vi "HFRR ADV v08.vi"() -> ()   [LabVIEW 2025] (continued)
        stop <- w5093 stop-if-true
        n3621 = local read "powstat"() -> (w5094:bool)
        n3622 = case shown="True" w5094 {
          frame False {
          }
          frame True {
            n3623 = local read "RUN"() -> (w5097:bool)
            n3624 = case shown="True" w5097 {
              frame False {
                w5127 = 65.0 ("y")
                n3625 = local read "Set Hz"() -> (w5155:dbl)
                n3626 = local read "NORMAL LOAD"() -> (w5156:dbl)
                n3627 = Multiply(x=w5155, y=60.0) -> (x*y=w5162:dbl)
                n3628 = Multiply(x=1.2 ("y"), y=0.949) -> (x*y=w5131:dbl)
                n3629 = Multiply(x=1.2 ("y"), y=0.8166) -> (x*y=w5135:dbl)
                n3630 = Multiply(x=1.2 ("y"), y=0.851) -> (x*y=w5130:dbl)
                n3631 = local read "FF 2"() -> (w5154:dbl)
                n3632 = Absolute Value(x=w5162) -> (abs(x)=w5160:dbl)
                n3633 = local read "Stroke"() -> (w5129:dbl)
                n3634 = Less?(x=w5129, y=w5135) -> (x < y?=w5132:bool)
                n3635 = In Range and Coerce(upper limit=w5131, x=w5129, lower limit=w5130) -> (In Range?=w5133:bool)  [unwired: 1 out]
                n3636 = case shown="13.." w5154 {
                  tunnel: [1 2 3] -> w5152
                  frame 0..10, Default {
                    # "Normal"
                  }
                  frame 11, 12 {
                  }
                  frame 13.. {
                  }
                }
                "FF STATE" <- w5152
                n3637 = local read "TEMP"() -> (w5115:dbl)
                n3638 = case shown="3601.." w5160 {
                  tunnel: [1 2 3] -> w5158
                  frame 0..3000, Default {
                    # "Normal"
                  }
                  frame 3001..3600 {
                  }
                  frame 3601.. {
                  }
                }
                n3639 = case shown="11.." w5156 {
                  tunnel: [1 3] -> w5157
                  frame 1..10, Default {
                  }
                  frame 11.. {
                  }
                }
                "NL STATE" <- w5157
                n3640 = Multiply(x=1.2 ("y"), y=0.95) -> (x*y=w5145:dbl)
                n3641 = Multiply(x=w5127, y=0.954) -> (x*y=w5119:dbl)
                n3642 = Or(x=w5132, y=w5133) -> (x .or. y?=w5134:bool)
                n3643 = Greater Or Equal?(x=w5129, y=w5145) -> (x >= y?=w5142:bool)
                n3644 = Multiply(x=w5127, y=0.99) -> (x*y=w5116:dbl)
                n3645 = Greater Or Equal?(x=w5115, y=w5116) -> (x >= y?=w5121:bool)
                n3646 = Greater Or Equal?(x=w5115, y=w5119) -> (x >= y?=w5118:bool)
                n3647 = case shown="0, 1, Default" w5129 {
                  tunnel: [1 3] -> w5146
                  frame 0, 1, Default {
                  }
                  frame 2.. {
                  }
                }
                n3648 = case shown="True" w5142 {
                  tunnel: [1 3] -> w5147
                  frame False {
                  }
                  frame True {
                  }
                }
                n3649 = case shown="True" w5134 {
                  tunnel: [1 2] -> w5148
                  frame False {
                  }
                  frame True {
                  }
                }
                n3650 = case shown="..0" w5115 {
                  tunnel: [2 3 3 1] -> w5122
                  frame 61, 62 {
                  }
                  frame 63.. {
                  }
                  frame ..0 {
                  }
                  frame 10..60, Default {
                  }
                }
                n3651 = case shown="True" w5121 {
                  tunnel: [1 3] -> w5123
                  frame False {
                  }
                  frame True {
                  }
                }
                n3652 = Number To Decimal String(number=w5158) -> (decimal integer string=w5159:string)  [unwired: 1 in]
                n3653 = case shown="True" w5118 {
                  tunnel: [1 2] -> w5124
                  frame False {
                  }
                  frame True {
                  }
                }
                n3654 = Number To Decimal String(number=1) -> (decimal integer string=→"Air temp":string)  [unwired: 1 in]
                n3655 = Number To Decimal String(number=w5152) -> (decimal integer string=→"ff_st":string)  [unwired: 1 in]
                n3656 = local write "sp_st"(w5159) -> ()
                n3657 = Number To Decimal String(number=w5157) -> (decimal integer string=→"nl_st":string)  [unwired: 1 in]
                n3658 = Build Array(w5122, w5123, w5124) -> (w5125:i32[])
                n3659 = Build Array(w5146, w5147, w5148) -> (w5149:i32[])
                n3660 = Array Max & Min(array=w5125) -> (max value=w5126:i32)  [unwired: 3 out]
                n3661 = Array Max & Min(array=w5149) -> (max value=w5150:i32)  [unwired: 3 out]
                n3662 = Number To Decimal String(number=w5126) -> (decimal integer string=w5114:string)  [unwired: 1 in]
                n3663 = Number To Decimal String(number=w5150) -> (decimal integer string=→"Stroke Ln 2":string)  [unwired: 1 in]
                n3664 = local write "temp_st"(w5114) -> ()
              }
              frame True {
                w5212 = 65.0 ("y")
                # "Healthy -1\nWarning -2\nError -3"
                n3665 = local read "TEMP"() -> (w5223:dbl)
                n3666 = local read "NORMAL LOAD"() -> (w5227:dbl)
                n3667 = local read "Set Hz"() -> (w5225:dbl)
                n3668 = Multiply(x=1.2 ("y"), y=0.949) -> (x*y=w5207:dbl)
                n3669 = Multiply(x=1.2 ("y"), y=0.8166) -> (x*y=w5203:dbl)
                n3670 = Multiply(x=1.2 ("y"), y=0.851) -> (x*y=w5208:dbl)
                n3671 = Multiply(x=w5212, y=0.954) -> (x*y=w5219:dbl)
                n3672 = Multiply(x=w5212, y=0.99) -> (x*y=w5222:dbl)
                n3673 = Greater Or Equal?(x=w5223, y=w5222) -> (x >= y?=w5217:bool)
                n3674 = Multiply(x=w5225, y=60.0) -> (x*y=w5231:dbl)
                n3675 = Greater Or Equal?(x=w5223, y=w5219) -> (x >= y?=w5220:bool)
                n3676 = local read "FF 2"() -> (w5226:dbl)
                n3677 = local read "Stroke"() -> (w5209:dbl)
                n3678 = Less?(x=w5209, y=w5203) -> (x < y?=w5206:bool)
                n3679 = In Range and Coerce(upper limit=w5207, x=w5209, lower limit=w5208) -> (In Range?=w5205:bool)  [unwired: 1 out]
                n3680 = Absolute Value(x=w5231) -> (abs(x)=w5229:dbl)
                n3681 = case shown="63.." w5223 {
                  tunnel: [2 3 3 1] -> w5216
                  frame 61, 62 {
                  }
                  frame 63.. {
                  }
                  frame ..0 {
                  }
                  frame 10..60, Default {
                  }
                }
                n3682 = case shown="True" w5217 {
                  tunnel: [1 3] -> w5215
                  frame False {
                  }
                  frame True {
                  }
                }
                n3683 = case shown="True" w5220 {
                  tunnel: [1 2] -> w5214
                  frame False {
                  }
                  frame True {
                  }
                }
                n3684 = Multiply(x=1.2 ("y"), y=0.95) -> (x*y=w5193:dbl)
                n3685 = case shown="1..10, Default" w5227 {
                  tunnel: [1 3] -> w5234
                  frame 1..10, Default {
                  }
                  frame 11.. {
                  }
                }
                n3686 = case shown="0..10, Default" w5226 {
                  tunnel: [1 2 3] -> w5233
                  frame 0..10, Default {
                  }
                  frame 11, 12 {
                  }
                  frame 13.. {
                  }
                }
                n3687 = case shown="3601.." w5229 {
                  tunnel: [1 2 3] -> w5228
                  frame 0..3000, Default {
                    # "Normal"
                  }
                  frame 3001..3600 {
                  }
                  frame 3601.. {
                  }
                }
                n3688 = Or(x=w5206, y=w5205) -> (x .or. y?=w5204:bool)
                n3689 = Greater Or Equal?(x=w5209, y=w5193) -> (x >= y?=w5196:bool)
                n3690 = case shown="0, 1, Default" w5209 {
                  tunnel: [1 3] -> w5192
                  frame 0, 1, Default {
                  }
                  frame 2.. {
                  }
                }
                n3691 = case shown="True" w5196 {
                  tunnel: [1 3] -> w5191
                  frame False {
                  }
                  frame True {
                  }
                }
                n3692 = case shown="True" w5204 {
                  tunnel: [1 2] -> w5190
                  frame False {
                  }
                  frame True {
                  }
                }
                n3693 = Build Array(w5216, w5215, w5214) -> (w5213:i32[])
                n3694 = Number To Decimal String(number=w5228) -> (decimal integer string=→"sp_st":string)  [unwired: 1 in]
                n3695 = Array Max & Min(array=w5213) -> (max value=w5210:i32)  [unwired: 3 out]
                "TEMP STATE" <- w5210
                n3696 = Number To Decimal String(number=w5234) -> (decimal integer string=w5237:string)  [unwired: 1 in]
                n3697 = Number To Decimal String(number=w5233) -> (decimal integer string=w5235:string)  [unwired: 1 in]
                n3698 = Number To Decimal String(number=w5210) -> (decimal integer string=→"temp_st":string)  [unwired: 1 in]
                n3699 = Build Array(w5192, w5191, w5190) -> (w5189:i32[])
                n3700 = local write "nl_st"(w5237) -> ()
                n3701 = local write "ff_st"(w5235) -> ()
                n3702 = Number To Decimal String(number=1) -> (decimal integer string=w5232:string)  [unwired: 1 in]
                n3703 = Array Max & Min(array=w5189) -> (max value=w5188:i32)  [unwired: 3 out]
                n3704 = local write "Air temp"(w5232) -> ()
                n3705 = Number To Decimal String(number=w5188) -> (decimal integer string=w5187:string)  [unwired: 1 in]
                n3706 = local write "Stroke Ln 2"(w5187) -> ()
              }
            }
            n3707 = local read "Stroke Ln 2"() -> (w5099:string)
            n3708 = local read "nl_st"() -> (w5105:string)
            n3709 = local read "ff_st"() -> (w5102:string)
            n3710 = local read "sp_st"() -> (w5103:string)
            n3711 = local read "temp_st"() -> (w5104:string)
            n3712 = local read "Air temp"() -> (w5098:string)
            n3713 = Replace Array Subset(array="in", new element #1=w5105, index #1=1 ("index"), new element #2=w5102, index #2=2 ("index"), new element #3=w5104, index #3=3 ("index"), new element #4=w5103, index #4=4 ("index"), new element #5=w5099, index #5=5 ("index"), new element #6=w5098, index #6=6 ("index"), new element #7="Sensor State" ("new element/subarray"), index #7=0 ("index")) -> (→"out":string[])
          }
        }
        n3714 = Wait (ms)(milliseconds to wait=u32 10) -> ()  [unwired: 1 out]
        n3715 = local read "Quit"() -> (w5093:bool)
      }
      n3716 = while {
        stop <- w5068 stop-if-true
        n3717 = local read "run replace"() -> (w5070:bool)
        n3718 = Wait (ms)(milliseconds to wait=u32 100) -> ()  [unwired: 1 out]
        n3719 = Equal?(x="FLAG 2", y=0.0) -> (x = y?=w5071:bool)
        n3720 = case shown="True" w5071 {
          frame False {
          }
          frame True {
            n3721 = local write "FLAG 2"(100.0 ("FLAG 2")) -> ()
            n3722 = call <vilib>:"Read Characters From File.vi"("file path (dialog if empty)"=path "C:/LAB-IQ-NXT/WO 2449 TT.sig", "convert eol? (no:F)"=FALSE ("append to file? (new file:F)")) -> ("character string"=w5074:string)  [unwired: 4 in, 3 out]
            n3723 = call <vilib>:"Read Characters From File.vi"("file path (dialog if empty)"=path "C:/LAB-IQ-NXT/WO 2449 TRH.sig", "convert eol? (no:F)"=FALSE ("append to file? (new file:F)")) -> ("character string"=w5075:string)  [unwired: 4 in, 3 out]
            n3724 = Decimal String To Number(string=w5074) -> (number=w5076:i32)  [unwired: 2 in, 1 out]
            n3725 = local write "Total No. of Tests"(w5076) -> ()
            n3726 = Decimal String To Number(string=w5075) -> (number=w5079:i32)  [unwired: 2 in, 1 out]
            n3727 = local write "SEN.RUN HRS"(w5079) -> ()
          }
        }
        n3728 = case shown="True" w5070 {
          frame False {
          }
          frame True {
            n3729 = Equal?(x="FLAG 4", y=0.0) -> (x = y?=w5083:bool)
            n3730 = case shown="False" w5083 {
              frame False {
                n3731 = Get Date/Time In Seconds() -> (seconds since 1Jan1904=w5089:timestamp)
                n3732 = local read "START 3"() -> (w5087:dbl)
                n3733 = To Double Precision Float(number=w5089) -> (double precision float=w5088:dbl)
                n3734 = Subtract(x=w5088, y=w5087) -> (x-y=→"SENSOR TIME":dbl)
              }
              frame True {
                n3735 = Get Date/Time In Seconds() -> (seconds since 1Jan1904=w5091:timestamp)
                n3736 = local write "FLAG 4"(100.0 ("FLAG")) -> ()
                n3737 = To Double Precision Float(number=w5091) -> (double precision float=→"START 3":dbl)
              }
            }
          }
        }
        n3738 = local read "Quit"() -> (w5068:bool)
      }
      n3739 = while {
        shift-right: [w4868] -> _
        shift-left: _ -> [w4869]
        tunnel: [w4864] -> _
        i -> [w4864]
        stop <- w4863 stop-if-true
        n3740 = Wait (ms)(milliseconds to wait=u32 50 ("Refresh Rate (ms)")) -> ()  [unwired: 1 out]
        n3741 = local read "Json End Flg"() -> (w4865:bool)
        n3742 = Not(x="Upld AR 2") -> ()  [unwired: 1 out]
        n3743 = local read "Upld AR 2"() -> (w4866:bool)
        n3744 = call "Elapsed Time9"("Time Target (s)"="Sen.Upload Rate (s)", "Reset"=FALSE, "Auto Reset"=TRUE) -> ("Time has Elapsed"=w4875:bool)  [unwired: 9 in, 7 out]
        n3745 = Or(x=w4875, y=w4865) -> (x .or. y?=w4871:bool)
        n3746 = case shown="True" w4871 {
          frame False {
          }
          frame True {
            w4967 = "\"SensorName\":\"" ("string")
            w4937 = " \"},{"
            w4962 = "\",\"SensorState\":\""
            w4964 = "\",\"SensorModelNumber\":\"" ("string")
            w4963 = "\",\"SensorRuntimeHours\":\"" ("string")
            n3747 = local read "model num"() -> (w4961:string[])
            n3748 = local read "Sensor name"() -> (w4980:string[])
            n3749 = local read "run"() -> (w4951:string[])
            n3750 = local read "SENSOR TIME"() -> (w4907:dbl)
            n3751 = local read "out"() -> (w4900:string[])
            n3752 = local read "Total No. of Tests"() -> (w4905:dbl)
            n3753 = Select(t=60.0, s="Run test 3", f=3600.0) -> (s? t:f=w4915:dbl)
            n3754 = Index Array(array=w4961, index #1=1 ("index")) -> (element #1=w4960:string, element #2=w4959:string, element #3=w4958:string, element #4=w4957:string, element #5=w4956:string, element #6=w4955:string)  [unwired: 5 in]
            n3755 = Index Array(array=w4951, index #1=1 ("index")) -> (element #1=w4950:string, element #2=w4949:string, element #3=w4948:string, element #4=w4947:string, element #5=w4946:string, element #6=w4945:string)  [unwired: 5 in]
            n3756 = Index Array(array=w4980, index #1=1 ("index")) -> (element #1=w4979:string, element #2=w4978:string, element #3=w4977:string, element #4=w4976:string, element #5=w4966:string, element #6=w4965:string)  [unwired: 5 in]
            n3757 = Index Array(array=w4900, index #1=1 ("index")) -> (element #1=w4932:string, element #2=w4931:string, element #3=w4930:string, element #4=w4929:string, element #5=w4928:string, element #6=w4927:string)  [unwired: 5 in]
            n3758 = local read "SEN.RUN HRS"() -> (w4903:dbl)
            n3759 = Divide(x=w4907, y=w4915) -> (x/y=w4914:dbl)
            n3760 = Increment(x=w4914) -> (x+1=w4910:dbl)
            n3761 = Number To Decimal String(number=w4910) -> (decimal integer string=→"run hrs":string)  [unwired: 1 in]
            n3762 = Divide(x=w4903, y=3600.0 ("f")) -> (x/y=w4898:dbl)
            n3763 = Round To Nearest(number=w4898) -> (nearest integer value=w4896:dbl)
            n3764 = Number To Decimal String(number=w4896) -> (decimal integer string=w4897:string)  [unwired: 1 in]
            n3765 = Number To Decimal String(number=w4905) -> (decimal integer string=w4906:string)  [unwired: 1 in]
            n3766 = local read "Model No"() -> (w4911:string)
            n3767 = local read "UUID"() -> (w5006:string)
            n3768 = local read "Serial No"() -> (w5010:string)
            n3769 = local read "Secret Key"() -> (w5011:string)
            n3770 = Concatenate Strings("\",\"MachineSerialNumber\":\"" ("string"), w5010) -> (w5014:string)
            n3771 = Concatenate Strings("\",\"ModelNumber\":\"" ("string"), w4911) -> (w4912:string)
            n3772 = Concatenate Strings("\",\"MachineRuntimeHours\":\"" ("string"), w4897) -> (w5015:string)
            n3773 = Concatenate Strings("\",\"MachineRuntimeCycles\":\"", w4906) -> (w5008:string)
            n3774 = Concatenate Strings(w4964, w4960) -> (w4994:string)
            n3775 = Concatenate Strings(w4963, w4950) -> (w4995:string)
            n3776 = Concatenate Strings(w4962, w4932) -> (w4993:string)
            n3777 = Concatenate Strings(w5014, w4912, w5015, w5008) -> (w5017:string)
            n3778 = Concatenate Strings(w4964, w4959) -> (w4991:string)
            n3779 = Concatenate Strings(w4963, w4949) -> (w4990:string)
            n3780 = Concatenate Strings(w4962, w4931) -> (w4992:string)
            n3781 = Concatenate Strings(w4964, w4958) -> (w4986:string)
            n3782 = Concatenate Strings(w4963, w4948) -> (w4987:string)
            n3783 = Concatenate Strings(w4962, w4930) -> (w4985:string)
            n3784 = Concatenate Strings(w4964, w4957) -> (w4983:string)
            n3785 = Concatenate Strings(w4963, w4947) -> (w4982:string)
            n3786 = Concatenate Strings(w4962, w4929) -> (w4984:string)
            n3787 = Concatenate Strings(w4994, w4995, w4993) -> (w4996:string)
            n3788 = Concatenate Strings(w4964, w4956) -> (w4973:string)
            n3789 = Concatenate Strings(w4963, w4946) -> (w4974:string)
            n3790 = Concatenate Strings(w4964, w4955) -> (w4970:string)
            n3791 = Concatenate Strings(w4963, w4945) -> (w4969:string)
            n3792 = Concatenate Strings(w4962, w4928) -> (w4972:string)
            n3793 = Concatenate Strings(w4962, w4927) -> (w4971:string)
            n3794 = Concatenate Strings("{\"SecretKey\":\"", w5011, w5017, "\",\"UUID\" : \"", w5006, "\",\"SensorInformation\":", "[{" ("string")) -> (w4944:string)
            n3795 = Concatenate Strings(w4991, w4990, w4992) -> (w4989:string)
            n3796 = Concatenate Strings(w4986, w4987, w4985) -> (w4988:string)
            n3797 = Concatenate Strings(w4983, w4982, w4984) -> (w4981:string)
            n3798 = Concatenate Strings(w4973, w4974, w4972) -> (w4975:string)
            n3799 = Concatenate Strings(w4970, w4969, w4971) -> (w4968:string)
            n3800 = Concatenate Strings(w4967, w4979, w4996, w4937) -> (w4943:string)
            n3801 = Concatenate Strings(w4967, w4978, w4989, w4937) -> (w4942:string)
            n3802 = Concatenate Strings(w4967, w4977, w4988, w4937) -> (w4941:string)
            n3803 = Concatenate Strings(w4967, w4976, w4981, w4937) -> (w4940:string)
            n3804 = Concatenate Strings(w4967, w4966, w4975, w4937) -> (w4939:string)
            n3805 = Concatenate Strings(w4967, w4965, w4968, "\"}" ("string")) -> (w4938:string)
            n3806 = Concatenate Strings(w4944, w4943, w4942, w4941, w4940, w4939, w4938, "]}" ("string")) -> (w4935:string)
            n3807 = local read "SEN.RUN HRS"() -> (w4902:dbl)
            n3808 = disable-structure shown="Disabled" {
              frame Disabled {
                n3809 = local read "state"() -> (w5021:string[])
                n3810 = Delete From Array(array=w5021, index=0) -> (array with subset deleted=w5019:string[])  [unwired: 1 in, 1 out]
                n3811 = for {
                  N: 6 -> [_]
                  tunnel: w5019 -> [w5032] mode=indexing
                  tunnel: [w5031] -> w5018 mode=indexing
                  n3812 = Equal?(x=w5032, y="Warning") -> (x = y?=w5028:bool)
                  n3813 = Equal?(x=w5032, y="Healthy") -> (x = y?=w5025:bool)
                  n3814 = Select(t="2" ("y"), s=w5028, f="3" ("y")) -> (s? t:f=w5023:string)
                  n3815 = Select(t="1" ("y"), s=w5025, f=w5023) -> (s? t:f=w5031:string)
                }
                "state1" <- w5018
              }
              frame Enabled {
              }
            }
            n3816 = stacked-sequence {
              tunnel: w4935 -> [w5043 _ _]
              tunnel: [_ _ w5059] -> _
              frame #0 {
                (unwired) FALSE ("convert eol (F)")
                w5045 = enum16{"start", "end", "current"}."start" ("pos mode (0:2)")
                n3817 = local read "Path"() -> (w5039:path)
                n3818 = Path To String(path=w5039) -> (string=w5051:string)
                n3819 = Concatenate Strings(w5051, "\\", "Sensor File Name") -> (w5052:string)
                n3820 = local write "standard output 2"(" ") -> ()
                n3821 = String To Path(string=w5052) -> (path=w5042:path)
                n3822 = call <vilib>:"Open_Create_Replace File.vi"("advisory dialog? (display:T)"=FALSE, "function (open:0)"=T24."create or replace", "file path"=w5042) -> ("error out"=w5055:errorcluster, "refnum"=w5054:refnum<file>)  [unwired: 5 in, 2 out]
                n3823 = Set File Position(refnum=w5054, from (0:start)=w5045, error in=w5055) -> (refnum out=w5035:refnum<file>, error out=w5034:errorcluster)  [unwired: 1 in]
                n3824 = Write to Binary File(file (use dialog)=w5035, data=" ", error in=w5034, 5:FALSE ("prepend array or string size? (T)")) -> (refnum out=w5046:refnum<file>, error out=w5047:errorcluster)  [unwired: 2 in, 1 out]
                n3825 = Set File Position(offset (in bytes) (0)=w5045, refnum=w5046, error in=w5047) -> (refnum out=w5038:refnum<file>, error out=w5037:errorcluster)  [unwired: 1 in]
                n3826 = Write to Binary File(file (use dialog)=w5038, data=w5043, error in=w5037, 5:FALSE ("prepend array or string size? (T)")) -> (error out=w5041:errorcluster)  [unwired: 2 in, 2 out]
                n3827 = flat-sequence {
                  tunnel: w5042 -> [w5057]
                  tunnel: w5041 -> [_]
                  frame #0 {
                    n3828 = call <vilib>:"Read Characters From File.vi"("file path (dialog if empty)"=w5057) -> ("character string"=→"Sensor Health JSON string":string)  [unwired: 5 in, 3 out]
                  }
                }
                "SinglePoint  2" <- w5043
              }
              frame #1 {
              }
              frame #2 {
                (unwired) "\"Stored\": true" ("string")
                n3829 = call <vilib>:"System Exec.vi"("run minimized? (F)"=TRUE, "wait until completion? (T)"=TRUE, "working directory"=path "C:/LAB-IQ-NXT", "command line"="C:\\LAB-IQ-NXT\\JPostH.bat") -> ("standard error"=→"Respose From Server 2":string, "standard output"=w5062:string)  [unwired: 4 in, 2 out]
                "standard output 2" <- w5062
                n3830 = Match Pattern(string=w5062, regular expression="JSONH Check String") -> (match substring=w5060:string, offset past match=w5059:i32)  [unwired: 1 in, 2 out]
                n3831 = Equal?(x=w5060, y="JSONH Check String") -> (x = y?=→"Upload \nConfirmed 2":bool)
              }
            }
            n3832 = Divide(x=w4902, y=3600.0 ("f")) -> (x/y=w4895:dbl)
            n3833 = local read "run time"() -> (w4952:string[])
            n3834 = Round To Nearest(number=w4895) -> (nearest integer value=w4894:dbl)
            n3835 = Number To Decimal String(number=w4894) -> (decimal integer string=w4893:string)  [unwired: 1 in]
            n3836 = Index Array(array="Sensor Information", index (col) #1=0 ("disabled index (col)"), index (col) #2=1 ("index (col)"), index (col) #3=2 ("index (col)"), index (col) #4=3 ("index (col)")) -> (element #1=→"Sensor name":string[], element #2=→"model num":string[], element #3=→"run time":string[], element #4=→"state":string[])  [unwired: 4 in]
            n3837 = Insert Into Array(array=w4952, index=1, new element #1=w4893, new element #2=w4893, new element #3=w4893, new element #4=w4893, new element #5=w4893, new element #6=w4893) -> (w4917:string[])
            "run" <- w4917
            n3838 = local read "out"() -> (w4899:string[])
            n3839 = local read "Sensor Information"() -> (w4919:string[][])
            n3840 = Replace Array Subset(array=w4919, new element #1=w4917, index (col) #1=2 ("disabled index (col)"), new element #2=w4899, index (col) #2=3 ("index (col)")) -> (w4918:string[][])  [unwired: 2 in]
            n3841 = local write "Sensor Information"(w4918) -> ()
          }
        }
        n3842 = case shown="True" w4866 {
          frame False {
          }
          frame True {
            n3843 = Equal?(x="FLAG", y=0.0) -> (x = y?=w4883:bool)
            n3844 = case shown="False" w4883 {
              frame False {
                n3845 = Get Date/Time In Seconds() -> (seconds since 1Jan1904=w4889:timestamp)
                n3846 = local read "START 2"() -> (w4887:dbl)
                n3847 = To Double Precision Float(number=w4889) -> (double precision float=w4888:dbl)
                n3848 = Subtract(x=w4888, y=w4887) -> (x-y=→"SENSOR TIME  2":dbl)
              }
              frame True {
                n3849 = Get Date/Time In Seconds() -> (seconds since 1Jan1904=w4891:timestamp)
                n3850 = To Double Precision Float(number=w4891) -> (double precision float=→"START 2":dbl)
                n3851 = local write "FLAG"(100.0 ("FLAG")) -> ()
              }
            }
          }
        }
        n3852 = disable-structure shown="Disabled" {
          disable-tunnel: w4869 -> [w4878 _]
          disable-tunnel: [w4877 _] -> w4868
          frame Disabled {
            n3853 = local read "Json St Flg"() -> (w4876:bool)
            n3854 = case shown="True" w4876 {
              tunnel: w4878 -> [w4879 w4881]
              tunnel: [w4879 w4880] -> w4877
              frame False {
              }
              frame True {
                n3855 = Increment(x=w4881) -> (x+1=w4880:dbl)
                "T cycle" <- w4880
                n3856 = local write "Json St Flg"(FALSE ("Json St Flg")) -> ()
              }
            }
          }
          frame Enabled {
          }
        }
        n3857 = local read "Quit"() -> (w4863:bool)
      }
    }
    frame Enabled {
    }
  }
  n3858 = stacked-sequence {
    tunnel: [w5261] -> w28
    frame #0 {
      w5261 = FALSE ("Upload \nConfirmed")
      n3859 = local write "Upload \nConfirmed"(w5261) -> ()
      n3860 = local write "St Str"("") -> ()
    }
  }
  n3861 = disable-structure shown="Disabled" {
    disable-tunnel: w28 -> [w5262 _]
    frame Disabled {
      n3862 = case shown="True" {
        selector: _ -> [_ _]
        tunnel: w5262 -> [_ w5263]
        frame False {
        }
        frame True {
          n3863 = while {
            tunnel: [w5269] -> _
            tunnel: w5263 -> [_]
            i -> [w5269]
            stop <- w5264 stop-if-true
            n3864 = local read "Json End Flg"() -> (w5268:bool)
            n3865 = Wait (ms)(milliseconds to wait=u32 20 ("Refresh Rate (ms)")) -> ()  [unwired: 1 out]
            n3866 = local read "refresh flag"() -> (w5265:bool)
            n3867 = local read "RUN"() -> (w5266:bool)
            n3868 = And(x=w5266, y=w5265) -> (x .and. y?=w5267:bool)
            n3869 = Or(x=w5267, y=w5268) -> (x .or. y?=w5270:bool)
            "AR Led" <- w5270
            n3870 = case shown="True" w5270 {
              frame False {
              }
              frame True {
                w5287 = "\",\""
                n3871 = local read "UUID"() -> (w5285:string)
                n3872 = local write "refresh flag"(FALSE ("refresh flag")) -> ()
                n3873 = local read "time"() -> (w5274:dbl)
                n3874 = Multiply(x=w5274, y=60.0) -> (x*y=w5273:dbl)
                n3875 = Concatenate Strings("UUID\" : \"", w5285, "\"}") -> (w5288:string)
                n3876 = Number To Fractional String(number=w5273, width (-)=i16 10, precision (6)=i16 4) -> (F-format string=w5302:string)  [unwired: 1 in]
                n3877 = Concatenate Strings("{", "\"Time\":\"", w5302, w5287) -> (w5297:string)
                n3878 = stacked-sequence {
                  tunnel: w5287 -> [w5350 w5358 w5365 w5373 w5381 w5390 w5397]
                  tunnel: [w5351 _ _ _ _ _ _] -> w5301
                  tunnel: [_ w5359 _ _ _ _ _] -> w5300
                  tunnel: [_ _ w5366 _ _ _ _] -> w5299
                  tunnel: [_ _ _ w5375 _ _ _] -> w5298
                  tunnel: w5288 -> [_ _ _ _ _ _ w5408]
                  tunnel: [_ _ _ _ _ _ w5407] -> w5284
                  tunnel: [_ _ _ _ _ w5387 _] -> w5283
                  tunnel: [_ _ _ _ w5380 _ _] -> w5282
                  frame #0 {
                    n3879 = local read "NORMAL LOAD"() -> (w5349:dbl)
                    n3880 = Number To Fractional String(number=w5349, width (-)=i16 10, precision (6)=i16 4) -> (F-format string=w5352:string)  [unwired: 1 in]
                    n3881 = Concatenate Strings("NormalLoad\":\"", w5352, w5350) -> (w5351:string)
                  }
                  frame #1 {
                    n3882 = local read "Temp"() -> (w5357:dbl)
                    n3883 = Number To Fractional String(number=w5357, width (-)=i16 10, precision (6)=i16 4) -> (F-format string=w5360:string)  [unwired: 1 in]
                    n3884 = Concatenate Strings("Temperature\":\"", w5360, w5358) -> (w5359:string)
                  }
                  frame #2 {
                    n3885 = local read "cof"() -> (w5363:dbl)
                    n3886 = Number To Fractional String(number=w5363, width (-)=i16 10, precision (6)=i16 4) -> (F-format string=w5367:string)  [unwired: 1 in]
                    n3887 = Concatenate Strings("FrictionalForce\":\"", w5367, w5365) -> (w5366:string)
                  }
                  frame #3 {
                    n3888 = local read "Set Hz"() -> (w5371:dbl)
                    n3889 = Multiply(x=w5371, y=60.0) -> (x*y=w5370:dbl)
                    n3890 = Number To Fractional String(number=w5370, width (-)=i16 10, precision (6)=i16 4) -> (F-format string=w5376:string)  [unwired: 1 in]
                    n3891 = Concatenate Strings("Speed\":\"", w5376, w5373) -> (w5375:string)
                  }
                  frame #4 {
                    n3892 = local read "Stroke Ln"() -> (w5379:dbl)
                    n3893 = Number To Fractional String(number=w5379, width (-)=i16 10, precision (6)=i16 4) -> (F-format string=w5383:string)  [unwired: 1 in]
                    n3894 = Concatenate Strings("LinearDeformation\":\"", w5383, w5381) -> (w5380:string)
                  }
                  frame #5 {
                    n3895 = local read "AIR TEMP"() -> (w5386:dbl)
                    n3896 = local read "Json St Flg"() -> (w5388:bool)
                    n3897 = local read "Json End Flg"() -> (w5389:bool)
                    n3898 = Number To Fractional String(number=w5386, width (-)=i16 10, precision (6)=i16 4) -> (F-format string=w5392:string)  [unwired: 1 in]
                    n3899 = Concatenate Strings("Vibration\":\"", w5392, w5390) -> (w5387:string)
                    n3900 = And(x=w5388, y=w5389) -> ()  [unwired: 1 out]
                  }
                  frame #6 {
                    n3901 = local read "Json End Flg"() -> (w5396:bool)
                    n3902 = Get Date/Time In Seconds() -> (seconds since 1Jan1904=w5404:timestamp)
                    n3903 = local read "Json St Flg"() -> (w5395:bool)
                    n3904 = To Double Precision Float(number=w5404) -> (double precision float=w5403:dbl)
                    n3905 = Subtract(x=w5403, y=2082844800.0) -> (x-y=w5401:dbl)
                    n3906 = Number To Fractional String(number=w5401, width (-)=i16 12, precision (6)=i16 0) -> (F-format string=w5398:string)  [unwired: 1 in]
                    n3907 = case shown="True" w5396 {
                      tunnel: ["" w5411] -> w5405
                      tunnel: w5398 -> [_ w5412]
                      tunnel: w5397 -> [_ w5410]
                      frame False {
                      }
                      frame True {
                        n3908 = local write "Json End Flg"(FALSE ("Json St Flg")) -> ()
                        n3909 = Concatenate Strings("End\": \"", w5412, w5410) -> (w5411:string)
                      }
                    }
                    n3910 = case shown="True" w5395 {
                      tunnel: [w5415 w5418] -> w5406
                      tunnel: w5398 -> [_ w5419]
                      tunnel: w5397 -> [_ w5416]
                      frame False {
                        n3911 = local read "St Str"() -> (w5415:string)
                      }
                      frame True {
                        n3912 = Concatenate Strings("Start\":\"", w5419, w5416) -> (w5418:string)
                        "St Str" <- w5418
                        n3913 = local write "Json St Flg"(FALSE ("Json St Flg")) -> ()
                      }
                    }
                    n3914 = Concatenate Strings(w5406, w5405, w5408) -> (w5407:string)
                  }
                }
                n3915 = local read "FILE"() -> (w5276:string)
                n3916 = Concatenate Strings("\",\"OperatorID\":\"" ("string"), "Operator ID") -> (w5279:string)
                n3917 = Concatenate Strings("\",\"DatasetTitle\":\"" ("string"), w5276) -> (w5278:string)
                n3918 = Concatenate Strings("\",\"SerialNumber\":\"" ("string"), "Serial No") -> (w5308:string)
                n3919 = Concatenate Strings("\",\"ModelNumber\":\"" ("string"), "Model No") -> (w5307:string)
                n3920 = Concatenate Strings(w5308, w5307) -> (w5290:string)
                n3921 = Concatenate Strings("{\"SecretKey\":\"", "Secret Key", w5290, w5279, w5278, "\",\"Samples\":[") -> (w5295:string)
                n3922 = Concatenate Strings(w5297, w5301, w5300, w5299, w5298, w5282, w5283, w5284) -> (w5296:string)
                n3923 = Concatenate Strings(w5295, w5296, "]}") -> (w5294:string)
                n3924 = stacked-sequence {
                  tunnel: w5294 -> [w5323 _ _]
                  tunnel: [_ _ w5340] -> _
                  frame #0 {
                    (unwired) FALSE ("convert eol (F)")
                    w5325 = enum16{"start", "end", "current"}."start" ("pos mode (0:2)")
                    n3925 = Path To String(path="Path") -> (string=w5331:string)
                    n3926 = Concatenate Strings(w5331, "\\", "Data File Name") -> (w5333:string)
                    n3927 = local write "standard output"(" ") -> ()
                    n3928 = String To Path(string=w5333) -> (path=w5322:path)
                    n3929 = call <vilib>:"Open_Create_Replace File.vi"("advisory dialog? (display:T)"=FALSE, "function (open:0)"=T24."create or replace", "file path"=w5322) -> ("error out"=w5336:errorcluster, "refnum"=w5335:refnum<file>)  [unwired: 5 in, 2 out]
                    n3930 = Set File Position(refnum=w5335, from (0:start)=w5325, error in=w5336) -> (refnum out=w5316:refnum<file>, error out=w5315:errorcluster)  [unwired: 1 in]
                    n3931 = Write to Binary File(file (use dialog)=w5316, data=" ", error in=w5315, 5:FALSE ("prepend array or string size? (T)")) -> (refnum out=w5326:refnum<file>, error out=w5327:errorcluster)  [unwired: 2 in, 1 out]
                    n3932 = Set File Position(offset (in bytes) (0)=w5325, refnum=w5326, error in=w5327) -> (refnum out=w5319:refnum<file>, error out=w5318:errorcluster)  [unwired: 1 in]
                    n3933 = Write to Binary File(file (use dialog)=w5319, data=w5323, error in=w5318, 5:FALSE ("prepend array or string size? (T)")) -> (error out=w5321:errorcluster)  [unwired: 2 in, 2 out]
                    n3934 = flat-sequence {
                      tunnel: w5322 -> [w5338]
                      tunnel: w5321 -> [_]
                      frame #0 {
                        n3935 = call <vilib>:"Read Characters From File.vi"("file path (dialog if empty)"=w5338) -> ("character string"=→"JSON string":string)  [unwired: 5 in, 3 out]
                      }
                    }
                    "SinglePoint" <- w5323
                  }
                  frame #1 {
                  }
                  frame #2 {
                    (unwired) "\"Stored\": true" ("string")
                    n3936 = call <vilib>:"System Exec.vi"("run minimized? (F)"=TRUE, "wait until completion? (T)"=TRUE, "working directory"=path "C:/LAB-IQ-NXT", "command line"="C:\\LAB-IQ-NXT\\JPost.bat") -> ("standard error"=→"Respose From Server":string, "standard output"=w5343:string)  [unwired: 4 in, 2 out]
                    "standard output" <- w5343
                    n3937 = Match Pattern(string=w5343, regular expression="JSON Check String") -> (match substring=w5341:string, offset past match=w5340:i32)  [unwired: 1 in, 2 out]
                    n3938 = Equal?(x=w5341, y="JSON Check String") -> (x = y?=→"Upload \nConfirmed":bool)
                  }
                }
              }
            }
            n3939 = local read "Quit"() -> (w5264:bool)
          }
        }
      }
    }
    frame Enabled {
    }
  }
  n3940 = disable-structure shown="Disabled" {
    disable-tunnel: _ -> [w5426 _]
    frame Disabled {
      n3941 = while {
        shift-right: [w5434] -> w5422
        shift-left: _ -> [w5435]
        shift-right: [w5432] -> w5423
        shift-left: errorcluster {"status"=TRUE, "code"=0, "source"="Init"} ("error out") -> [w5433]
        shift-right: [w5430] -> _
        shift-left: "" -> [w5431]
        tunnel: [w5428] -> _
        tunnel: w5426 -> [_]
        i -> [w5428]
        stop <- w5427 stop-if-true
        n3942 = flat-sequence {
          tunnel: [w5436] -> w5429
          frame #0 {
            n3943 = Wait (ms)(milliseconds to wait=10.0 ("Delay")) -> (millisecond timer value=w5436:u32)
          }
        }
        n3944 = case shown="No Error" w5433 {
          selector: w5433 -> [w5469 w5591]
          tunnel: [w5451 w5593] -> w5434
          tunnel: [w5450 w5592] -> w5432
          tunnel: w5435 -> [w5470 w5585]
          tunnel: w5431 -> [w5449 w5584]
          tunnel: [w5448 w5584] -> w5430
          tunnel: w5429 -> [_ _]
          frame No Error {
            n3945 = Concatenate Strings("COMMAND", "\r", "\n") -> (w5460:string)
            n3946 = case shown="True" "Measure" {
              tunnel: w5470 -> [w5496 w5503]
              tunnel: w5469 -> [w5495 w5502]
              tunnel: [w5496 w5501] -> w5468
              tunnel: [w5495 w5500] -> w5447
              tunnel: w5460 -> [_ w5499]
              frame False {
              }
              frame True {
                n3947 = VISA Write(VISA resource name=w5503, write buffer=w5499, error in (no error)=w5502) -> (VISA resource name out=w5501:refnum<visa-resource-name>, error out=w5500:errorcluster)  [unwired: 1 out]
                n3948 = local write "Read String"("") -> ()
                n3949 = local write "Measure"(FALSE) -> ()
              }
            }
            n3950 = property class="Instr"(reference=w5468, error in=w5447) -> (reference out=w5467:refnum<visa-resource-name>, error out=w5466:errorcluster, "Serial Settings:Number of Bytes at Serial Port"=w5465:u32)
            n3951 = Greater?(x=w5465, y=u32 100) -> (0:w5463:bool)
            n3952 = case shown="True" w5463 {
              tunnel: w5467 -> [w5506 w5531]
              tunnel: w5466 -> [w5505 w5530]
              tunnel: w5465 -> [_ w5529]
              tunnel: [w5506 w5528] -> w5453
              tunnel: [w5505 w5527] -> w5452
              tunnel: w5449 -> [w5504 w5526]
              tunnel: [w5504 ""] -> w5448
              frame False {
              }
              frame True {
                w5516 = u32 6 ("y")
                # "Page 84 of \nmanual"
                n3953 = VISA Read(VISA resource name=w5531, byte count=w5529, error in (no error)=w5530) -> (VISA resource name out=w5528:refnum<visa-resource-name>, read buffer=w5524:string, error out=w5527:errorcluster)  [unwired: 1 out]
                n3954 = while {
                  tunnel: w5524 -> [w5580]
                  tunnel: [w5576] -> w5518 mode=indexing
                  tunnel: [w5570] -> w5522 mode=indexing
                  tunnel: [w5568] -> _
                  i -> [w5568]
                  stop <- w5573 stop-if-true
                  n3955 = String Subset(string=w5580, offset (0)=w5568) -> (substring=w5575:string)  [unwired: 1 in]
                  n3956 = String To Byte Array(string=w5575) -> (unsigned byte array=w5579:u8[])
                  n3957 = String Length(string=w5575) -> (length=w5574:i32)
                  n3958 = Index Array(array=w5579) -> (element=w5578:u8)  [unwired: 1 in]
                  n3959 = Equal To 0?(x=w5574) -> (x = 0?=w5573:bool)
                  n3960 = Number To Boolean Array(number=w5578) -> (Boolean array=w5572:bool[])
                  n3961 = Reverse 1D Array(array=w5572) -> (reversed array=w5571:bool[])
                  n3962 = And(x=w5572, y=bool[] [FALSE, FALSE, FALSE, FALSE, FALSE, FALSE, TRUE, TRUE] ("Boolean array")) -> (x .and. y?=w5576:bool[])
                  n3963 = And(x=w5571, y=bool[] [FALSE, FALSE, TRUE, TRUE, TRUE, TRUE, TRUE, TRUE] ("Boolean array")) -> (x .and. y?=w5570:bool[])
                }
                n3964 = Concatenate Strings(w5526, w5524) -> (→"Read String":string)
                n3965 = while {
                  tunnel: w5518 -> [w5567] mode=indexing
                  tunnel: [w5563] -> w5521
                  i -> [w5563]
                  stop <- w5564 stop-if-true
                  n3966 = Search 1D Array(1D array=w5567, element=TRUE) -> (index of element=w5565:i32)  [unwired: 1 in]
                  n3967 = Less Than 0?(x=w5565) -> (x < 0?=w5564:bool)
                }
                n3968 = Delete From Array(array=w5522, length=w5521, index (row)=0) -> (array with subset deleted=w5517:bool[][])  [unwired: 1 in, 1 out]
                n3969 = Array Size(array=w5517) -> (size(s)=w5519:i32[])
                n3970 = Index Array(array=w5519) -> (element=w5511:i32)  [unwired: 1 in]
                n3971 = Greater?(x=w5511, y=w5516) -> (0:w5514:bool)
                n3972 = Subtract(x=w5511, y=w5516) -> (x-y=w5515:u32)
                n3973 = Select(t=w5515, s=w5514, f=u32 0) -> (s? t:f=w5512:u32)
                n3974 = while {
                  tunnel: w5517 -> [w5550]
                  tunnel: [w5552] -> w5510 mode=indexing
                  tunnel: w5512 -> [w5534]
                  i -> [w5551]
                  stop <- w5549 stop-if-true
                  w5541 = 6 ("index")
                  w5540 = 2 ("length")
                  # "Page 65 of \nmanual"
                  n3975 = Multiply(x=u32 3 ("y"), y=w5551) -> (x*y=w5548:u32)
                  n3976 = Divide(x=u32 102 ("y"), y=u32 65520) -> (x/y=w5558:dbl)
                  n3977 = Greater Or Equal?(x=w5548, y=w5534) -> (x >= y?=w5549:bool)
                  n3978 = Index Array(array=w5550, index (row) #1=w5548) -> (element #1=w5546:bool[], element #2=w5545:bool[], element #3=w5544:bool[])  [unwired: 5 in]
                  n3979 = Reverse 1D Array(array=w5546) -> (reversed array=w5539:bool[])
                  n3980 = Reverse 1D Array(array=w5545) -> (reversed array=w5543:bool[])
                  n3981 = Reverse 1D Array(array=w5544) -> (reversed array=w5542:bool[])
                  n3982 = Delete From Array(array=w5539, length=w5540, index=w5541) -> (array with subset deleted=w5535:bool[])  [unwired: 1 out]
                  n3983 = Delete From Array(array=w5543, length=w5540, index=w5541) -> (array with subset deleted=w5536:bool[])  [unwired: 1 out]
                  n3984 = Delete From Array(array=w5542, length=w5540, index=w5541) -> (array with subset deleted=w5537:bool[])  [unwired: 1 out]
                  n3985 = Insert Into Array(array=bool[] [] ("Boolean array"), new element #1=w5535, new element #2=w5536, new element #3=w5537) -> (w5538:bool[])  [unwired: 1 in]
                  n3986 = Boolean Array To Number(Boolean array=w5538) -> (number=w5547:u32)
                  n3987 = Multiply(x=w5558, y=w5547) -> (x*y=w5557:dbl)
                  n3988 = Decrement(x=w5557) -> (x-1=w5556:dbl)
                  n3989 = Divide(x=w5556, y=u32 100) -> (x/y=w5554:dbl)
                  n3990 = Multiply(x=w5554, y=u32 10) -> (x*y=w5552:dbl)
                }
                n3991 = Delete From Array(array=w5510) -> (array with subset deleted=w5509:dbl[])  [unwired: 2 in, 1 out]
                "Waveform Graph 5" <- w5509
                "Waveform Chart 3" <- w5509
                n3992 = call-poly <vilib>:"Mean.vi"("X"=w5509) -> ("mean"=w5508:dbl)  [unwired: 1 out]
                "Measure_LDS" <- w5508
                n3993 = case shown="True" "Zero 4" {
                  tunnel: w5508 -> [_ w5533]
                  frame False {
                  }
                  frame True {
                    n3994 = local write "Zero 4"(FALSE ("Zero 4")) -> ()
                    "z_measure" <- w5533
                  }
                }
              }
            }
            n3995 = local read "Measure_LDS"() -> (w5443:dbl)
            n3996 = local read "Disp (mm)"() -> (w5442:dbl)
            n3997 = local read "Boolean 7"() -> (w5441:bool)
            n3998 = local read "Boolean 8"() -> (w5440:bool)
            n3999 = case shown="True" "Boolean 8" {
              tunnel: w5442 -> [_ w5473]
              tunnel: w5443 -> [_ w5472]
              frame False {
              }
              frame True {
                n4000 = local read "Captured Values 2"() -> (w5476:dbl[][])
                n4001 = Build Array(w5473, w5472) -> (w5471:dbl[])
                n4002 = Build Array (concatenate)(w5476, w5471) -> (w5474:dbl[][])
                n4003 = local write "Captured Values 2"(w5474) -> ()
                n4004 = local write "Boolean 8"(FALSE ("Boolean 8")) -> ()
              }
            }
            n4005 = call "Build XY Graph"("Enable"=w5440, "Reset"=w5441, "Y Input"=w5443, "X Input"=w5442) -> ("XY Graph"=→"?":cluster{"Y":dbl[], "Y":dbl[]}[])  [unwired: 6 in, 1 out]
            n4006 = case shown="True" "Boolean 9" {
              frame False {
              }
              frame True {
                n4007 = local read "Captured Values 2"() -> (w5478:dbl[][])
                n4008 = Index Array(array=w5478, index (col) #1=0 ("disabled index (col)"), index (col) #2=1 ("index (col)")) -> (element #1=w5481:dbl[], element #2=w5480:dbl[])  [unwired: 2 in]
                n4009 = call <vilib>:"Linear Fit.vi"("Y"=w5481, "X"=w5480) -> ("slope"=→"Slope":dbl, "intercept"=→"Intercept":dbl)  [unwired: 9 in, 3 out]
                n4010 = local write "Boolean 9"(FALSE ("Boolean 9")) -> ()
              }
            }
            n4011 = case shown="True" "Boolean 7" {
              frame False {
              }
              frame True {
                n4012 = local write "Captured Values 2"(dbl[][] [] ("Captured Values")) -> ()
                n4013 = local write "Boolean 7"(FALSE ("Boolean 7")) -> ()
              }
            }
            n4014 = Concatenate Strings("COMMAND 2", "\r", "\n") -> (w5455:string)
            n4015 = case shown="True" "Measure 2" {
              tunnel: w5453 -> [w5488 w5494]
              tunnel: w5452 -> [w5487 w5493]
              tunnel: [w5488 w5492] -> w5451
              tunnel: [w5487 w5491] -> w5450
              tunnel: w5455 -> [_ w5490]
              frame False {
              }
              frame True {
                n4016 = local write "Measure 2"(FALSE ("WRITE")) -> ()
                n4017 = VISA Write(VISA resource name=w5494, write buffer=w5490, error in (no error)=w5493) -> (VISA resource name out=w5492:refnum<visa-resource-name>, error out=w5491:errorcluster)  [unwired: 1 out]
              }
            }
          }
          frame Error {
            w5583 = u16 10 items=["1.0"=10, "1.5"=15, "2.0"=20] ("stop bits (10: 1 bit)")
            n4018 = Wait (ms)(milliseconds to wait=u32 20) -> ()  [unwired: 1 out]
            n4019 = VISA Close(VISA resource name=w5585, error in (no error)=w5591) -> (error out=w5590:errorcluster)
            n4020 = call <vilib>:"Clear Errors.vi"("error in (no error)"=w5590) -> ("error out"=w5589:errorcluster)  [unwired: 5 in, 1 out]
            n4021 = call-poly "VISA Configure Serial Port"("VISA resource name"="Laser Disp Sensor", "timeout (10sec)"=u32 200, "Enable Termination\nChar (T)"=TRUE ("Enable Termination\nChar (T)"), "baud rate (9600)"=u32 921600, "error in (no error)"=w5589, "stop bits (10: 1 bit)"=w5583) -> ("VISA resource name out"=w5593:refnum<visa-resource-name>, "error out"=w5592:errorcluster)  [unwired: 8 in]
          }
        }
        n4022 = local read "Quit"() -> (w5427:bool)
      }
      n4023 = VISA Close(VISA resource name=w5422, error in (no error)=w5423) -> (error out=w5421:errorcluster)
      n4024 = call <vilib>:"Clear Errors.vi"("error in (no error)"=w5421) -> ()  [unwired: 5 in, 2 out]
    }
    frame Enabled {
    }
  }
  n4025 = disable-structure shown="Disabled" {
    disable-tunnel: _ -> [w5598 _]
    frame Disabled {
      n4026 = while {
        tunnel: [w5605] -> _
        shift-right: [w5602] -> w5595
        shift-left: _ -> [w5604]
        shift-right: [w5603] -> w5596
        shift-left: errorcluster {"status"=TRUE, "code"=0, "source"="Init"} ("error out") -> [w5601]
        tunnel: w5598 -> [_]
        i -> [w5605]
        stop <- w5599 stop-if-true
        n4027 = flat-sequence {
          tunnel: w5601 -> [w5696]
          tunnel: [w5696] -> w5600
          frame #0 {
            n4028 = Wait (ms)(milliseconds to wait=u32 50) -> ()  [unwired: 1 out]
          }
        }
        n4029 = case shown="No Error" w5600 {
          selector: w5600 -> [w5646 w5689]
          tunnel: w5604 -> [w5645 w5688]
          tunnel: [w5612 w5679] -> w5603
          tunnel: [w5613 w5687] -> w5602
          frame No Error {
            w5639 = T25 {"Mode"=enum."RTU", "Slave Address"=1} ("Serial Parameters")
            n4030 = call-poly <vilib>:"MB Serial Master Query (poly).vi"("VISA resource name"=w5645, "Starting Address"=i16 1000, "Quantity"=u16 1, "Timeout"=u32 1000, "error in"=w5646, "Serial Parameters"=w5639) -> ("VISA resource name out"=w5640:refnum<visa-resource-name>, "Input Registers"=w5642:u16[], "error out"=w5638:errorcluster)  [unwired: 10 in, 1 out]
            n4031 = Random Number (0-1)() -> (number: 0 to 1=w5627:dbl)
            n4032 = Index Array(array=w5642, index=0) -> (element=w5637:u16)
            n4033 = Subtract(x=w5627, y=0.5) -> (x-y=w5626:dbl)
            n4034 = Divide(x=w5637, y=10 ("index")) -> (x/y=w5631:dbl)
            n4035 = Multiply(x=w5626, y=0.5) -> (x*y=w5625:dbl)
            n4036 = Add(x=w5631, y=w5625) -> (x+y=w5630:dbl)
            n4037 = local read "Amb temp"() -> (w5614:dbl)
            n4038 = Multiply(x=w5630, y=0.2) -> (x*y=w5634:dbl)
            n4039 = Multiply(x=w5614, y=0.8) -> (x*y=w5632:dbl)
            n4040 = Add(x=w5634, y=w5632) -> (x+y=w5615:dbl)
            n4041 = local read "set temp old"() -> (w5609:dbl)
            n4042 = local write "Amb temp"(w5615) -> ()
            n4043 = Select(t="SetTemp 2", s="Heater", f=100.0) -> (s? t:f=w5610:dbl)
            n4044 = Not Equal?(x=w5610, y=w5609) -> (x != y?=w5608:bool)
            n4045 = case shown="True" w5608 {
              tunnel: w5640 -> [w5674 w5676]
              tunnel: [w5673 w5676] -> w5620
              tunnel: w5638 -> [w5672 w5675]
              tunnel: [w5671 w5675] -> w5618
              tunnel: w5610 -> [w5666 _]
              tunnel: w5639 -> [w5668 w5677]
              tunnel: [w5668 w5677] -> w5621
              frame True {
                n4046 = Multiply(x=w5666, y=10 ("index")) -> (x*y=w5665:dbl)
                n4047 = call-poly <vilib>:"MB Serial Master Query (poly).vi"("VISA resource name"=w5674, "Address"=u16 0, "Holding Register"=w5665, "Timeout"=u32 1000, "error in"=w5672, "Serial Parameters"=w5668) -> ("VISA resource name out"=w5673:refnum<visa-resource-name>, "error out"=w5671:errorcluster)  [unwired: 11 in, 1 out]
                "set temp old" <- w5666
              }
              frame False {
              }
            }
            n4048 = flat-sequence {
              tunnel: [w5647] -> _
              tunnel: [w5647] -> w5617
              tunnel: w5618 -> [w5647]
              frame #0 {
                n4049 = Wait (ms)(milliseconds to wait=u32 100) -> ()  [unwired: 1 out]
              }
            }
            n4050 = call "Elapsed Time12"("Time Target (s)"=2.0, "Auto Reset"=TRUE) -> ("Time has Elapsed"=w5622:bool)  [unwired: 10 in, 7 out]
            n4051 = case shown="True" w5622 {
              tunnel: w5621 -> [w5651 w5664]
              tunnel: [w5651 w5664] -> _
              tunnel: [w5650 w5662] -> w5613
              tunnel: w5620 -> [w5650 w5663]
              tunnel: [w5649 w5660] -> w5612
              tunnel: w5617 -> [w5649 w5661]
              frame False {
              }
              frame True {
                n4052 = call-poly <vilib>:"MB Serial Master Query (poly).vi"("VISA resource name"=w5663, "Starting Address"=i16 1003 ("Addr"), "Quantity"=u16 1, "Timeout"=u32 1000, "error in"=w5661, "Serial Parameters"=w5664) -> ("VISA resource name out"=w5662:refnum<visa-resource-name>, "Input Registers"=w5657:u16[], "error out"=w5660:errorcluster)  [unwired: 10 in, 1 out]
                n4053 = Index Array(array=w5657, index=0) -> (element=w5656:u16)
                n4054 = Divide(x=w5656, y=u16 10) -> (x/y=w5652:dbl)
                n4055 = local write "set temp old"(w5652) -> ()
                n4056 = local write "SetTemp"(w5652) -> ()
              }
            }
            "Error Code" <- w5612
            n4057 = Unbundle(w5612) -> ("status"=→"TK4 status":bool)  [unwired: 2 out]
            "SetTemp" <- "SetTemp 2"
          }
          frame Error {
            w5691 = u16 0 items=["None", "Odd", "Even", "Mark", "Space"] ("Parity")
            w5692 = u16 0 items=["None", "XON/XOFF", "RTS/CTS", "XON/XOFF & RTS/CTS", "DTR/DSR", "XON/XOFF & DTR/DSR"] ("Flow Control")
            n4058 = VISA Clear(VISA resource name=w5688, error in (no error)=w5689) -> (VISA resource name out=w5682:refnum<visa-resource-name>, error out=w5680:errorcluster)
            n4059 = VISA Close(VISA resource name=w5682, error in (no error)=w5680) -> (error out=w5681:errorcluster)
            n4060 = call <vilib>:"Clear Errors.vi"("error in (no error)"=w5681) -> ("error out"=w5690:errorcluster)  [unwired: 5 in, 1 out]
            n4061 = Unbundle By Name(T25 {"Mode"=enum."RTU", "Slave Address"=1} ("input cluster")) -> ("Mode"=w5693:enum16{"RTU", "ASCII"})
